vi "Read Kitchen.vi"(8 "error in (no error)":errorcluster, 11 "COOKING in":refnum<class "COOKING.lvclass">) -> (0 "error out":errorcluster, 2 "Kitchen":refnum<class "Message Enqueuer.lvclass">, 3 "COOKING out":refnum<class "COOKING.lvclass">)   [LabVIEW 2021, in "Chef States.lvlib" / "COOKING.lvclass"]
uses:
  COOKING.lvclass
  <vilib>/ActorFramework/Message Enqueuer/Message Enqueuer.lvclass
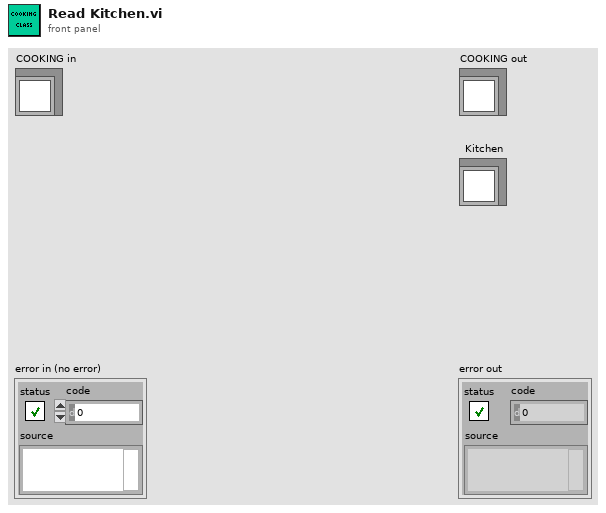
[diagram p1: front panel]
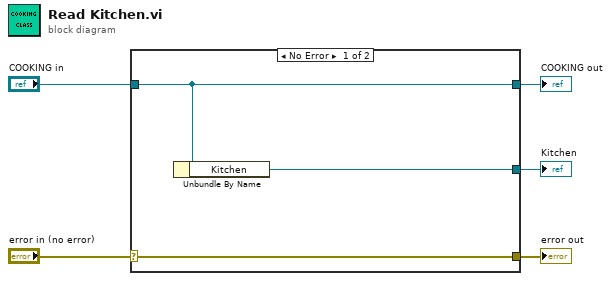
[diagram p0: block diagram]
diagram:
  n1 = case shown="No Error" "error in (no error)" {
    selector: "error in (no error)" -> [w8 w9]
    tunnel: [w8 w9] -> w4
    tunnel: [w7 w10] -> w2
    tunnel: "COOKING in" -> [w7 w10]
    tunnel: [w6 _] -> w1
    frame No Error {
      n2 = Unbundle By Name(w7) -> ("Kitchen"=w6:refnum<class "Message Enqueuer.lvclass">)
    }
    frame Error {
    }
  }
  "error out" <- w4
  "COOKING out" <- w2
  "Kitchen" <- w1
